vi "SelectDataElectNameXY.vi"(0 "dsc_board_address":string, 5 "elec_num":string, 7 "area_name":string, 11 "错误输入":errorcluster) -> (3 "area_name":string, 4 "detec_elec_name_mapx_mapy":string[](array[string]), 6 "detec_electrode_name":string, 8 "electrodes_map_x":string, 10 "electrodes_map_y":string, 15 "error out":errorcluster)   [LabVIEW 2014]
uses:
  DataBase.lvlib
  DetectElecrodes/DetectElectros.lvlib
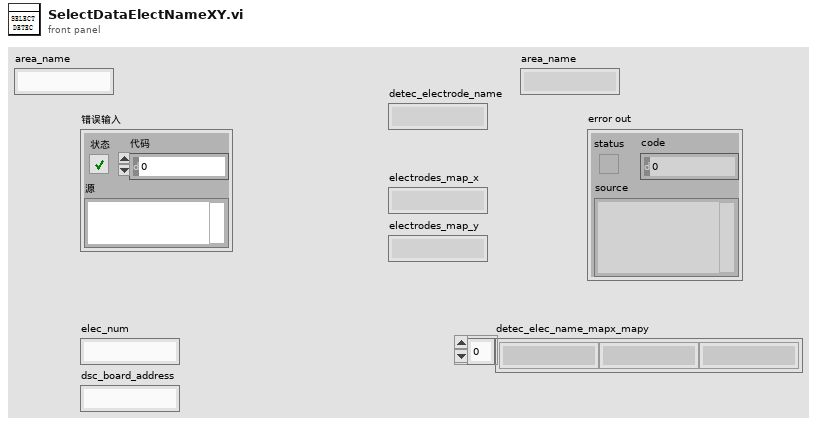
[diagram p1: front panel]
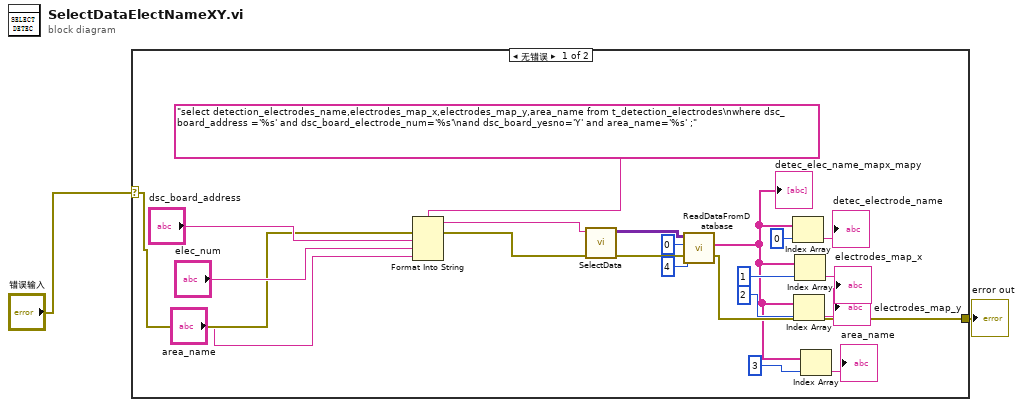
[diagram p0: block diagram]
diagram:
  n1 = case shown="无错误" "错误输入" {
    selector: "错误输入" -> [w11 w23]
    tunnel: [w12 w23] -> w2
    frame No Error {
      n2 = Format Into String(format string="select detection_electrodes_name,electrodes_map_x,electrodes_map_y,area_name from t_detection_electrodes\nwhere dsc_board_address ='%s' and dsc_board_electrode_num='%s'\nand dsc_board_yesno='Y' and area_name='%s' ;", error in=w11, "dsc_board_address", "elec_num", "area_name") -> (resulting string=w21:string, error out=w20:errorcluster)  [unwired: 1 in]
      n3 = call "SelectData.vi"("SQL query"=w21, "error in"=w20) -> ("recordset data"=w17:variant[][], "error out"=w12:errorcluster)  [unwired: 6 in]
      n4 = call "ReadDataFromDatabase.vi"("长度"=4, "index"=0, "recordset data"=w17) -> ("一行记录"=w5:string[])  [unwired: 7 in, 1 out]
      "detec_elec_name_mapx_mapy" <- w5
      n5 = Index Array(array=w5, index=0 ("索引")) -> (element=→"detec_electrode_name":string)
      n6 = Index Array(array=w5, index=2 ("索引")) -> (element=→"electrodes_map_y":string)
      n7 = Index Array(array=w5, index=1 ("索引")) -> (element=→"electrodes_map_x":string)
      n8 = Index Array(array=w5, index=3 ("索引")) -> (element=→"area_name":string)
    }
    frame Error {
    }
  }
  "error out" <- w2
